vi "Bridge Sim InpZ.vi"(0 "f [Hz]":dbl format="%#_6p") -> (5 "aperture":dbl, 6 "Cp":dbl format="%#_6p", 8 "Gp":dbl format="%#_6p", 9 "fs":dbl)   [LabVIEW 2020]
doc: "Simulate input impedance calibration measurement."
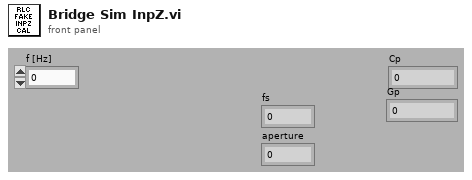
[diagram p1: front panel]
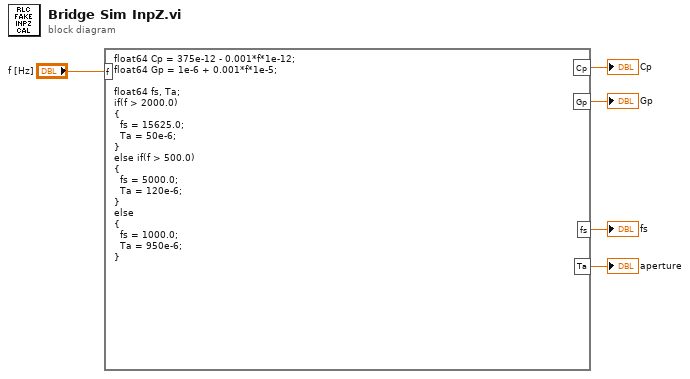
[diagram p0: block diagram]
diagram:
  n1 = formula code="float64 Cp = 375e-12 - 0.001*f*1e-12;\nfloat64 Gp = 1e-6 + 0.001*f*1e-5;\n\nfloat64 fs, Ta;\nif(f > 2000.0)\n{\n  fs = 15625.0;\n  Ta = 50e-6;\n}\nelse if(f > 500.0)\n{\n  fs = 5000.0;\n  Ta = 120e-6;\n}\nelse\n{\n  fs = 1000.0;\n  Ta = 950e-6;\n}"("f"="f [Hz]") -> ("Cp"=→"Cp":dbl, "Gp"=→"Gp":dbl, "fs"=→"fs":dbl, "Ta"=→"aperture":dbl)
